vi "Strain array to data.vi"(8 "Error In":errorcluster, 10 "Strain array":u8[](array[numeric])) -> (0 "Error Out":errorcluster, 2 "Strain data":T1)   [LabVIEW 2016]
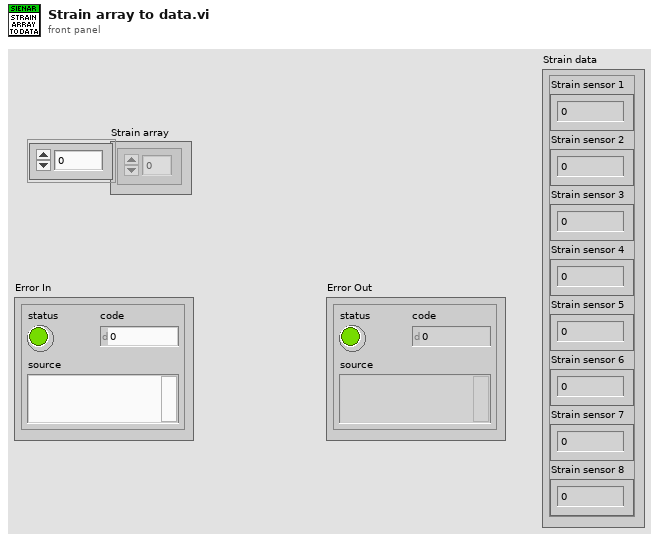
[diagram p1: front panel]
types:
  T1 = cluster{"Strain sensor 1":sgl, "Strain sensor 2":sgl, "Strain sensor 3":sgl, "Strain sensor 4":sgl, "Strain sensor 5":sgl, "Strain sensor 6":sgl, "Strain sensor 7":sgl, "Strain sensor 8":sgl}
  T2 = cluster{"[0]":dbl, "[1]":dbl, "[2]":dbl, "[3]":dbl, "[4]":dbl, "[5]":dbl, "[6]":dbl, "[7]":dbl}
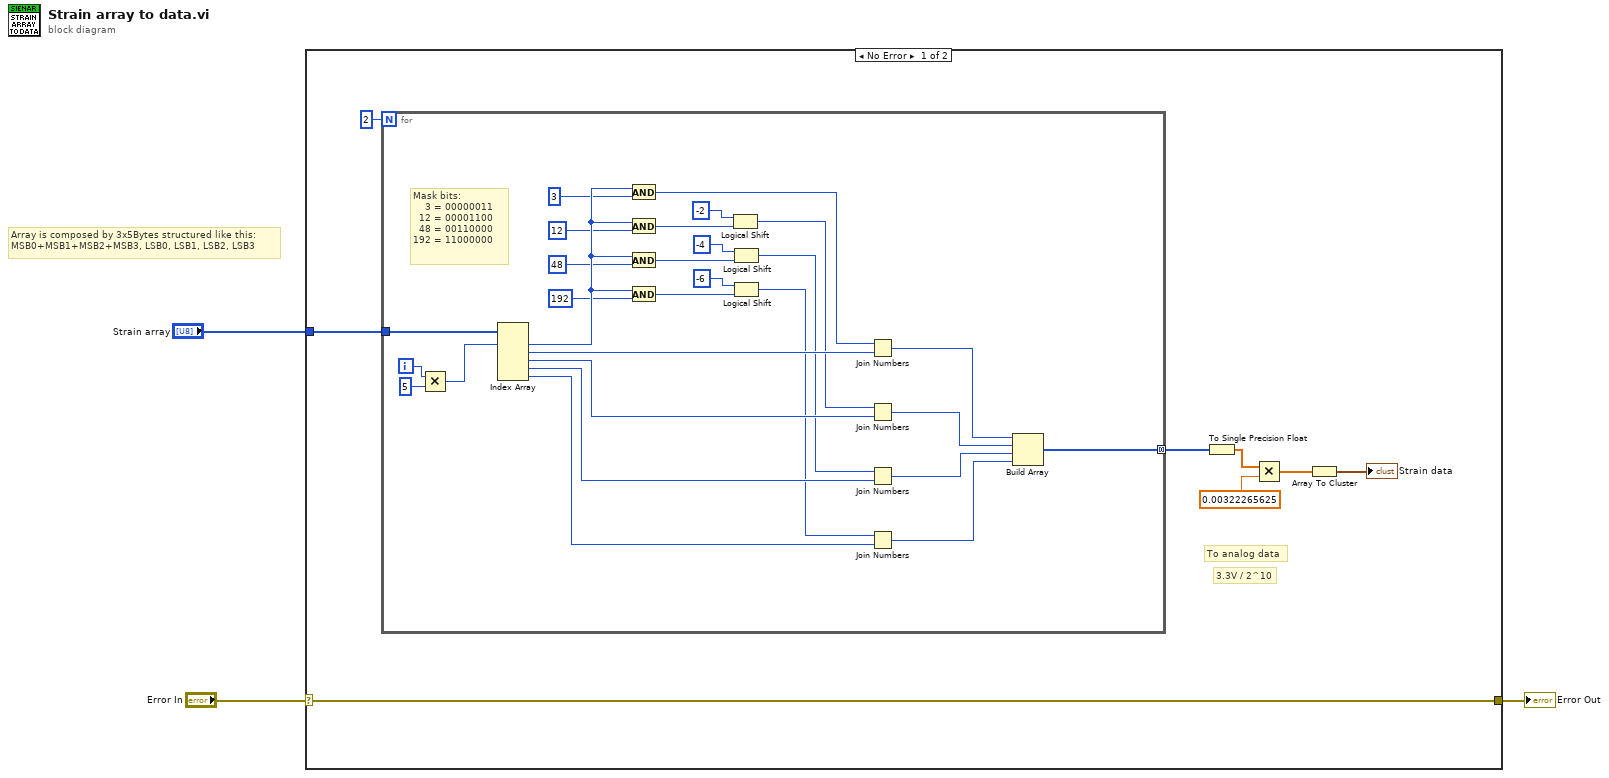
[diagram p0: block diagram]
diagram:
  # "Array is composed by 3x5Bytes structured like this: \nMSB0+MSB1+MSB2+MSB3, LSB0, LSB1, LSB2, LSB3"
  n1 = case shown="No Error" "Error In" {
    selector: "Error In" -> [w9 w40]
    tunnel: "Strain array" -> [w10 _]
    tunnel: [w9 w40] -> w1
    frame No Error {
      # "3.3V / 2^10"
      # "To analog data"
      n2 = for {
        N: 2 -> [_]
        tunnel: w10 -> [w39]
        tunnel: [w12] -> w8 mode=concatenating
        i -> [w38]
        # "Mask bits:\n    3 = 00000011\n  12 = 00001100\n  48 = 00110000\n192 = 11000000"
        n3 = Multiply(x=w38, y=5) -> (x*y=w36:i32)
        n4 = Index Array(array=w39, index #1=w36) -> (element #1=w35:u8, element #2=w24:u8, element #3=w22:u8, element #4=w19:u8, element #5=w17:u8)  [unwired: 4 in]
        n5 = And(x=w35, y=u8 3) -> (x .and. y?=w23:u8)
        n6 = And(x=w35, y=u8 12) -> (x .and. y?=w30:u8)
        n7 = And(x=w35, y=u8 48) -> (x .and. y?=w27:u8)
        n8 = And(x=w35, y=u8 192) -> (x .and. y?=w25:u8)
        n9 = Logical Shift(y=i16 -2, x=w30) -> (x << y=w21:u8)
        n10 = Logical Shift(y=i16 -4, x=w27) -> (x << y=w20:u8)
        n11 = Logical Shift(y=i16 -6, x=w25) -> (x << y=w18:u8)
        n12 = Join Numbers(hi=w23, lo=w24) -> ((hi.lo)=w16:u16)
        n13 = Join Numbers(hi=w21, lo=w22) -> ((hi.lo)=w15:u16)
        n14 = Join Numbers(hi=w20, lo=w19) -> ((hi.lo)=w14:u16)
        n15 = Join Numbers(hi=w18, lo=w17) -> ((hi.lo)=w13:u16)
        n16 = Build Array(w16, w15, w14, w13) -> (w12:u16[])
      }
      n17 = To Single Precision Float(number=w8) -> (single precision float=w4:sgl[])
      n18 = Multiply(x=w4, y=0.00322265625) -> (x*y=w7:dbl[])
      n19 = Array To Cluster(array=w7) -> (cluster=→"Strain data":T2)
    }
    frame Error {
    }
  }
  "Error Out" <- w1
